vi "Read Pre-measurement cycling.vi"(11 "PIC-Device in":refnum<class "PIC-Device.lvclass">) -> (2 "Pre-measurement cycling":T1={"Cycle"=FALSE, "Number of cycles"=2000, "Cycles Executed"=0}, 3 "PIC-Device out":refnum<class "PIC-Device.lvclass">)   [LabVIEW 2020, in "PIC-Device.lvclass"]
uses:
  PIC-Device.lvclass
  PIC-Device.lvclass/PIC-Device.ctl
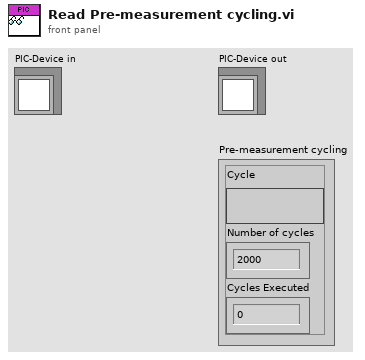
[diagram p1: front panel]
types:
  T1 = cluster{"Cycle":bool, "Number of cycles":u32, "Cycles Executed":u32}
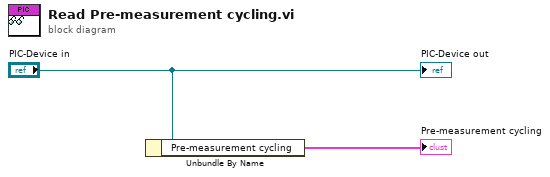
[diagram p0: block diagram]
diagram:
  n1 = Unbundle By Name("PIC-Device in") -> ("Pre-measurement cycling"=→"Pre-measurement cycling":T1)
  "PIC-Device out" <- "PIC-Device in"
